vi "Next Chart Name.vi"(8 "error in (no error)":errorcluster, 11 "Historian Charting Manager in":refnum<class "Historian Charting Manager.lvclass">) -> (0 "error out":errorcluster, 2 "Next Chart Num":i32, 3 "Historian Charting Manager out":refnum<class "Historian Charting Manager.lvclass">)   [LabVIEW 2020, in "VolatusGUI.lvlib" / "Historian Charting Manager.lvclass"]
uses:
  Historian Charting Manager.lvclass
  Historian Charting Manager.lvclass/Historian Charting Manager.ctl
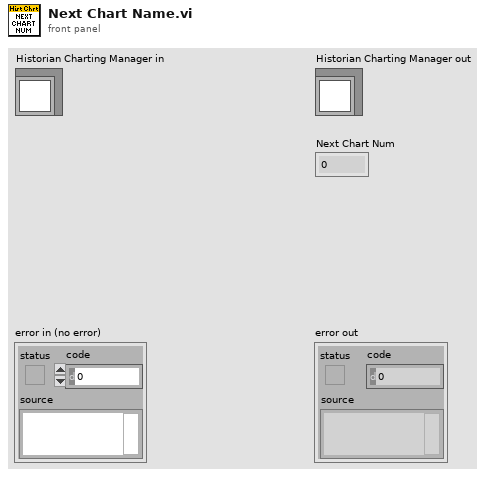
[diagram p1: front panel]
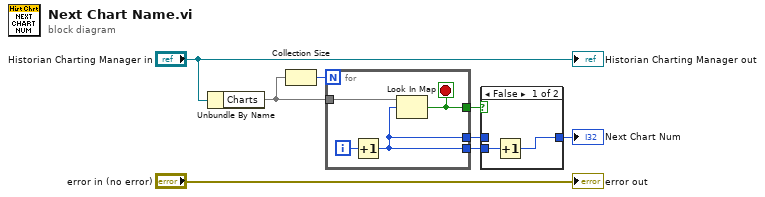
[diagram p0: block diagram]
diagram:
  n1 = Unbundle By Name("Historian Charting Manager in") -> ("Charts"=w2:map{i32, refnum<class "MessageQ.lvclass">})
  n2 = Collection Size(1:w2) -> (0:w6:i32)
  n3 = for {
    N: w6 -> [_]
    tunnel: w2 -> [w11]
    tunnel: [w9] -> w4
    tunnel: [w10] -> w5
    tunnel: [w9] -> w3
    i -> [w12]
    stop <- w10 stop-if-true
    n4 = Increment(x=w12) -> (x+1=w9:i32)
    n5 = Look In Map(map=w11, key=w9) -> (key not found?=w10:bool)  [unwired: 1 in, 1 out]
  }
  n6 = case shown="False" w5 {
    tunnel: w4 -> [_ w15]
    tunnel: w3 -> [w14 _]
    tunnel: [w13 w15] -> w1
    frame False {
      n7 = Increment(x=w14) -> (x+1=w13:i32)
    }
    frame True {
    }
  }
  "Next Chart Num" <- w1
  "error out" <- "error in (no error)"
  "Historian Charting Manager out" <- "Historian Charting Manager in"
